vi "Rd Wr Script Defaults.vi"(8 "error in (no error)":errorcluster, 10 "Write? (F:Read)":bool, 11 "Script Settings":T1) -> (0 "error out":errorcluster, 3 "Script Settings":T1)   [LabVIEW 2021]
uses:
  CC cluster Script Panel Defaults.ctl
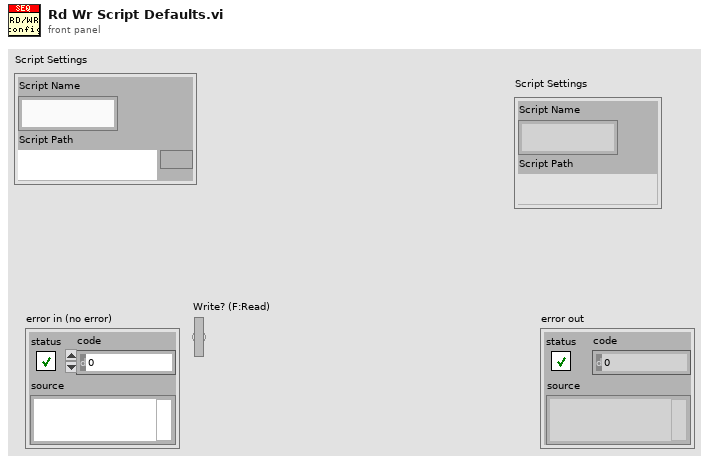
[diagram p1: front panel]
types:
  T1 = typedef "CC cluster Script Panel Defaults.ctl" = cluster{"Script Name":string, "Script Path":path}
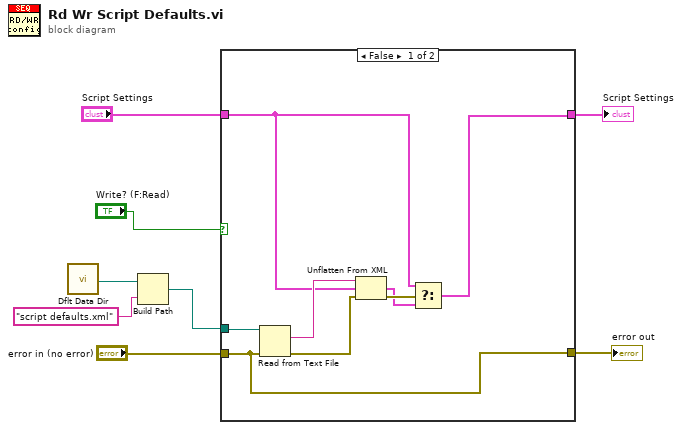
[diagram p0: block diagram]
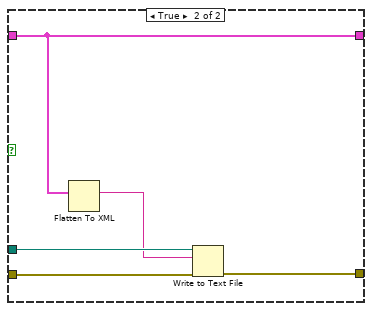
[diagram p2: hidden frame]
diagram:
  n1 = call <vilib>:"Dflt Data Dir.vi"() -> ("App:Default Data Directory"=w5:path)
  n2 = Build Path(base path=w5, name or relative path="script defaults.xml") -> (appended path=w4:path)
  n3 = case shown="False" "Write? (F:Read)" {
    tunnel: "error in (no error)" -> [w9 w21]
    tunnel: "Script Settings" -> [w12 w17]
    tunnel: w4 -> [w16 w20]
    tunnel: [w9 w18] -> w3
    tunnel: [w10 w17] -> w2
    frame False {
      n4 = Read from Text File(file (use dialog)=w16, error in=w9) -> (text=w15:string, error out=w14:errorcluster)  [unwired: 2 in, 2 out]
      n5 = Unflatten From XML(xml string=w15, type=w12, error in (no error)=w14) -> (value=w11:T1, error out=w13:errorcluster)
      n6 = Select(t=w12, s=w13, f=w11) -> (s? t:f=w10:T1)
    }
    frame True {
      n7 = Flatten To XML(6:w17) -> (2:w19:string)
      n8 = Write to Text File(file (use dialog)=w20, text=w19, error in=w21) -> (error out=w18:errorcluster)  [unwired: 1 in, 2 out]
    }
  }
  "error out" <- w3
  "Script Settings" <- w2
